vi "Facade 1.vi"(0 "Data In":T5, 2 "Display State In":T3, 3 "Container State":T4) -> (6 "Data Out":T5, 7 "Display State Out":T3, 8 "Action":T2)   [LabVIEW 2016, in "ZebraTable.lvlib" / "XControl 1.xctl"]
uses:
  XControl 1.xctl
  Data 1.ctl
  <vilib>/_xctls/Container State.ctl
  State 1.ctl
  <vilib>/_xctls/Action.ctl
  <vilib>/Utility/miscctls.llb/LVBoundsTypeDef.ctl
  <vilib>/_xctls/XControlSupport.lvlib
panel:
  out "XControl:Container Bounds":T1
  out "ALL vi":string[][](table)
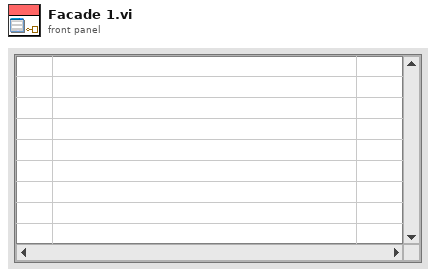
[diagram p1: front panel]
types:
  T1 = typedef "LVBoundsTypeDef.ctl" = cluster{"Width":u32, "Height":u32}
  T2 = typedef "XControlSupport.lvlib/Action.ctl" = cluster{"Data Changed?":bool, "State Changed?":bool, "Action Name":string}
  T3 = typedef "ZebraTable.lvlib/XControl 1.xctl/State 1.ctl" = cluster{"Color Box":u32}
  T4 = typedef "XControlSupport.lvlib/Container State.ctl" = cluster{"Indicator?":bool, "Run Mode?":bool, " Refnum":refnum<vi>}
  T5 = typedef "ZebraTable.lvlib/XControl 1.xctl/Data 1.ctl" = string[][]
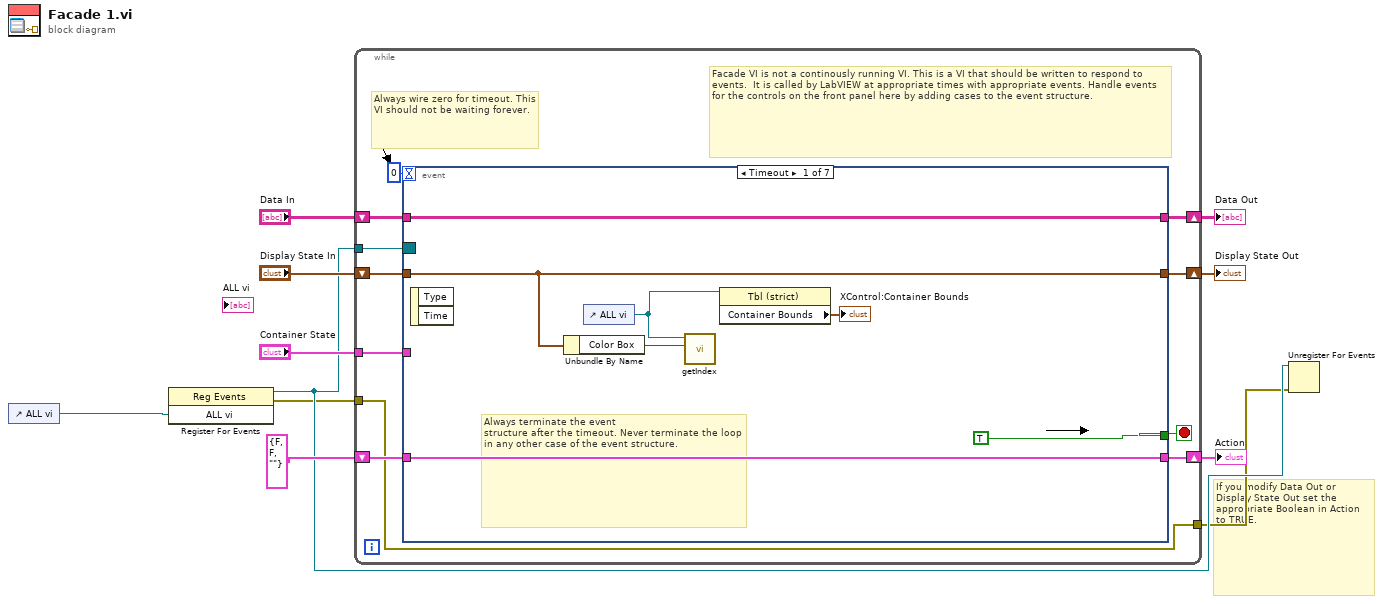
[diagram p0: block diagram]
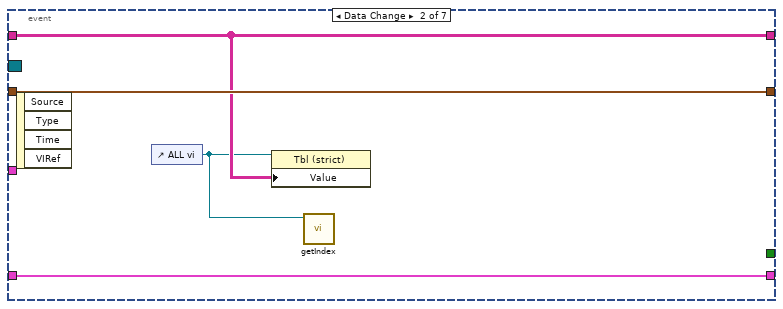
[diagram p2: hidden frame]
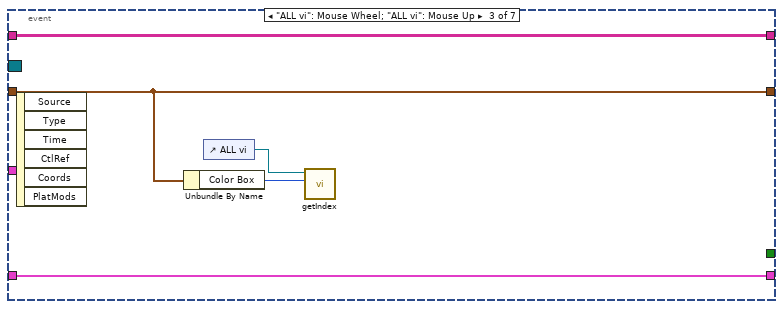
[diagram p3: hidden frame]
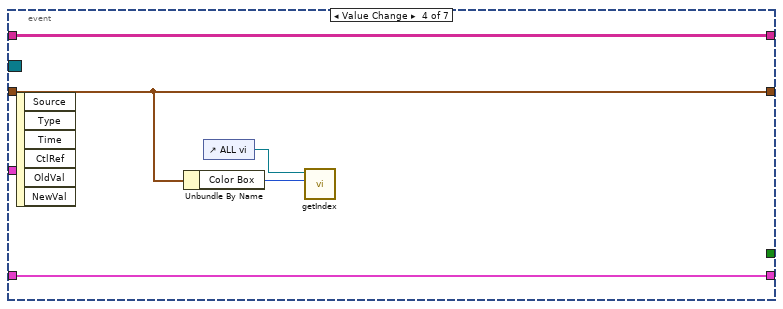
[diagram p4: hidden frame]
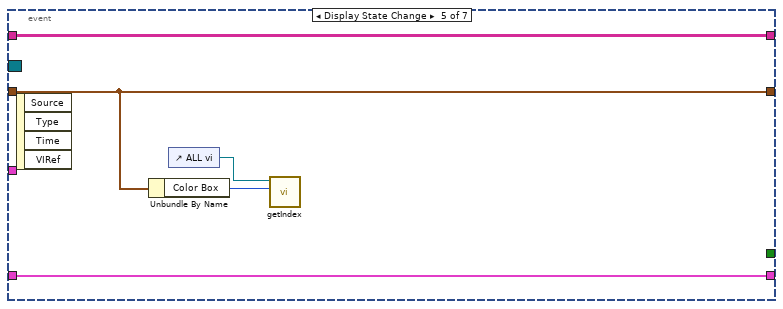
[diagram p5: hidden frame]
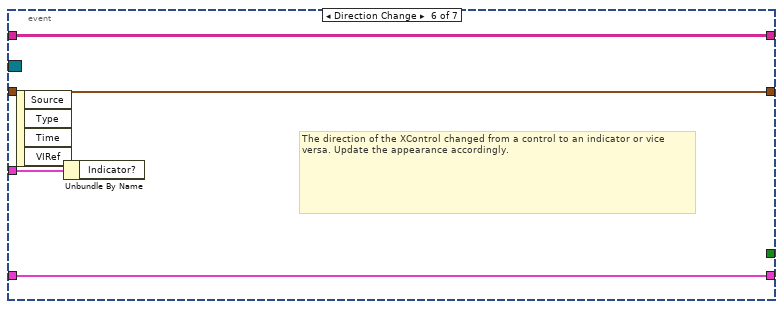
[diagram p6: hidden frame]
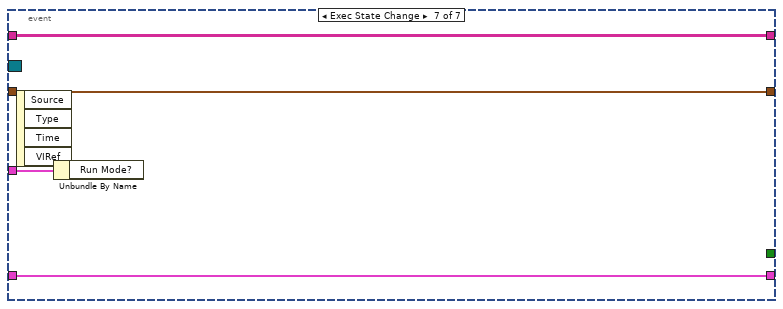
[diagram p7: hidden frame]
diagram:
  # "If you modify Data Out or\nDisplay State Out set the\nappropriate Boolean in Action\nto TRUE."
  n1 = control-ref of="ALL vi"() -> (w1:refnum<vi>)
  n2 = register-events(w1) -> (reference out=w4:refnum<event-registration>, error out=w3:errorcluster)  [unwired: 2 in]
  n3 = while {
    shift-right: [w21] -> w8
    shift-left: "Display State In" -> [w22]
    tunnel: "Container State" -> [w18]
    shift-right: [w16] -> w11
    shift-left: "Data In" -> [w17]
    shift-right: [w14] -> w6
    shift-left: T2 {"Data Changed?"=FALSE, "State Changed?"=FALSE, "Action Name"=""} ("Action") -> [w15]
    tunnel: w4 -> [w13]
    tunnel: [w12] -> w2
    tunnel: w3 -> [w12]
    stop <- w20 stop-if-true
    # "Facade VI is not a continously running VI. This is a VI that should be written to respond to events.  It is called by LabVIEW at appropriate times with appropriate events. Handle events for the controls on the front panel here by adding cases to the event structure."
    # "Always wire zero for timeout. This\nVI should not be waiting forever."
    n4 = event shown="[0] Timeout" {
      selector: w13 -> [_ _ _ _ _ _ _]
      dyn-events: _ -> [_ _ _ _ _ _ _]
      timeout: 0 -> [_ _ _ _ _ _ _]
      tunnel: w22 -> [w25 w33 w35 w40 w44 w51 w53]
      tunnel: [w25 w33 w35 w40 w44 w51 w53] -> w21
      tunnel: [TRUE _ _ _ _ _ _] -> w20
      tunnel: w18 -> [_ _ _ _ _ w52 w56]
      tunnel: w17 -> [w27 w31 w37 w42 w48 w50 w55]
      tunnel: [w27 w31 w37 w42 w48 w50 w55] -> w16
      tunnel: [w28 w32 w38 w43 w47 w49 w54] -> w14
      tunnel: w15 -> [w28 w32 w38 w43 w47 w49 w54]
      event Timeout {
        # "Always terminate the event\nstructure after the timeout. Never terminate the loop in any other case of the event structure."
        n5 = event-data() -> ()  [unwired: 1 in, 2 out]
        n6 = Unbundle By Name(w25) -> ("Color Box"=w26:u32)
        n7 = control-ref of="ALL vi"() -> (w24:refnum<vi>)
        n8 = call "getIndex.vi"("Active Cell:Cell Background Color"=w26, "TableRef"=w24) -> ()  [unwired: 9 in, 1 out]
        n9 = property class="Tbl (strict)"(reference=w24) -> ("Container Bounds"=→"XControl:Container Bounds":T1)  [unwired: 1 in, 2 out]
      }
      event Data Change {
        n10 = event-data() -> ()  [unwired: 1 in, 4 out]
        n11 = control-ref of="ALL vi"() -> (w30:refnum<vi>)
        n12 = property class="Tbl (strict)"(reference=w30, "Value"=w31) -> ()  [unwired: 1 in, 2 out]
        n13 = call "getIndex.vi"("TableRef"=w30) -> ()  [unwired: 10 in, 1 out]
      }
      event "ALL vi": Mouse Wheel; "ALL vi": Mouse Up {
        n14 = event-data() -> ()  [unwired: 1 in, 6 out]
        n15 = Unbundle By Name(w35) -> ("Color Box"=w34:u32)
        n16 = control-ref of="ALL vi"() -> (w36:refnum<vi>)
        n17 = call "getIndex.vi"("Active Cell:Cell Background Color"=w34, "TableRef"=w36) -> ()  [unwired: 9 in, 1 out]
      }
      event Value Change {
        n18 = event-data() -> ()  [unwired: 1 in, 6 out]
        n19 = Unbundle By Name(w40) -> ("Color Box"=w39:u32)
        n20 = control-ref of="ALL vi"() -> (w41:refnum<vi>)
        n21 = call "getIndex.vi"("Active Cell:Cell Background Color"=w39, "TableRef"=w41) -> ()  [unwired: 9 in, 1 out]
      }
      event Display State Change {
        n22 = event-data() -> ()  [unwired: 1 in, 4 out]
        n23 = Unbundle By Name(w44) -> ("Color Box"=w45:u32)
        n24 = control-ref of="ALL vi"() -> (w46:refnum<vi>)
        n25 = call "getIndex.vi"("Active Cell:Cell Background Color"=w45, "TableRef"=w46) -> ()  [unwired: 9 in, 1 out]
      }
      event Direction Change {
        # "The direction of the XControl changed from a control to an indicator or vice versa. Update the appearance accordingly."
        n26 = event-data() -> ()  [unwired: 1 in, 4 out]
        n27 = Unbundle By Name(w52) -> ()  [unwired: 1 out]
      }
      event Exec State Change {
        n28 = event-data() -> ()  [unwired: 1 in, 4 out]
        n29 = Unbundle By Name(w56) -> ()  [unwired: 1 out]
      }
    }
  }
  "Display State Out" <- w8
  "Data Out" <- w11
  "Action" <- w6
  n30 = Unregister For Events(event registration refnum=w4, error in=w2) -> ()  [unwired: 1 out]
